vi "License Activator.vi"(8 "error constant":errorcluster) -> (0 "error out":errorcluster)   [LabVIEW 2019]
panel:
  out "Iso Activated":bool
  out "UCT Activated":bool
  out "Sat Activated":bool
  out "Consol Activated":bool
  out "Permea Activated":bool
  out "Shear Activated":bool
  out "TUU Activated":bool
  out "TS Activated":bool
  in  "Iso Generate":bool
  in  "UCT Generate":bool
  in  "Sat Generate":bool
  in  "Cons Generate":bool
  in  "Permeability Generate":bool
  in  "Shearbox Generate":bool
  in  "TUU Generate":bool
  in  "TS Generate":bool
  in  "Isotropic Consolidation":string
  in  "UCT":string
  in  "Saturation (Incremental)":string
  in  "Consolidation (Stepped Loadning/Swelling)":string
  in  "Permeability":string
  in  "Shearbox":string
  in  "Triaxial UU":string
  in  "Triaxial Shear":string
  # "Test Type Module"
  # "Activation Code"
  # "Action"
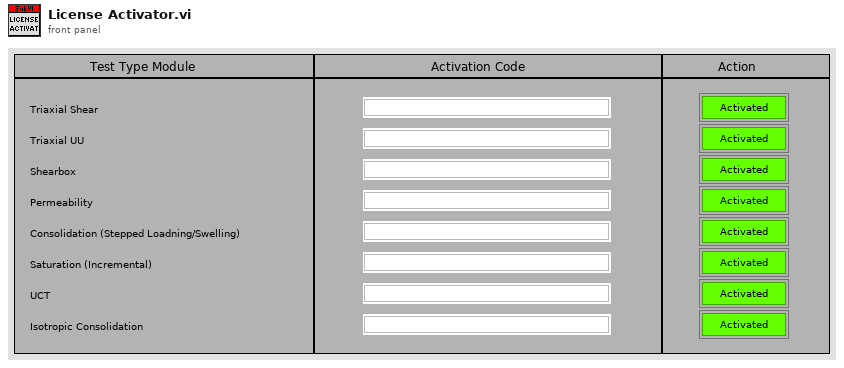
[diagram p1: front panel]
types:
  T1 = enum16{"open", "replace", "create", "open or create", "replace or create", "replace or create with confirmation"}
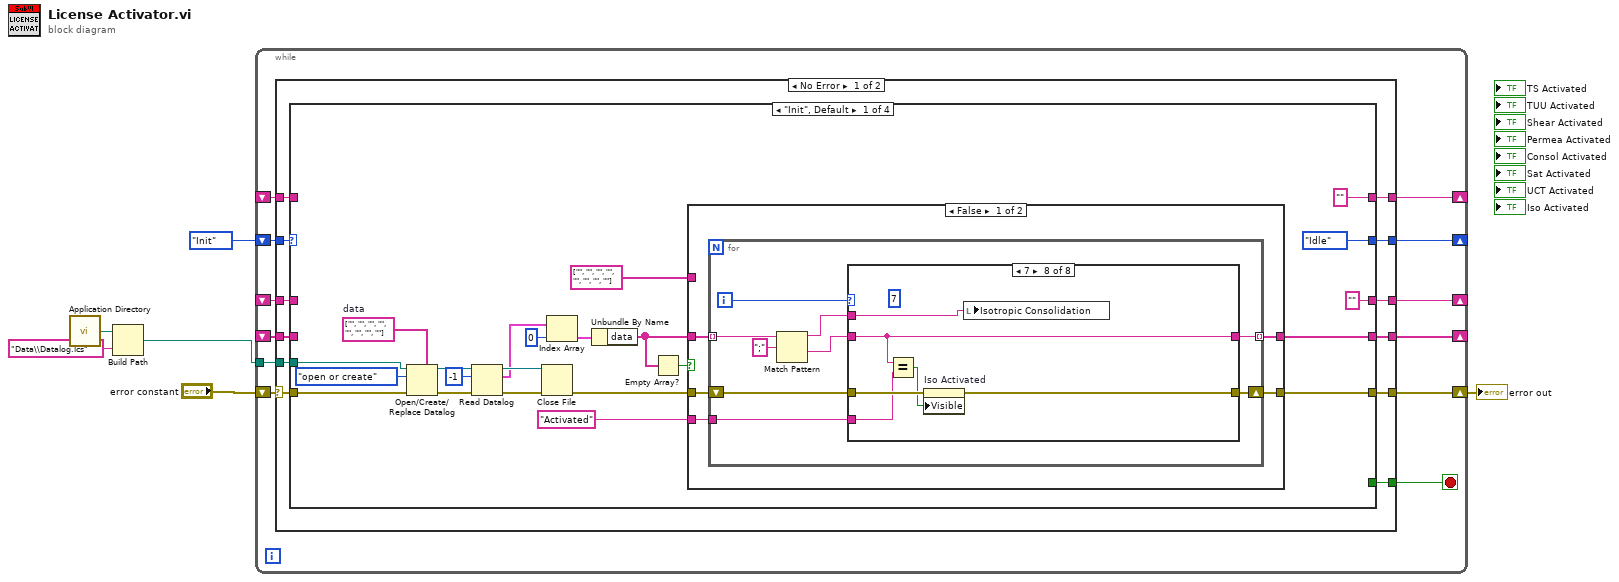
[diagram p0: block diagram]
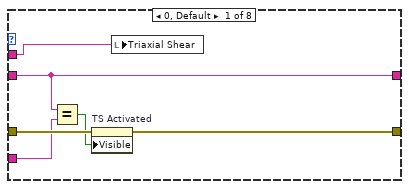
[diagram p2: hidden frame]
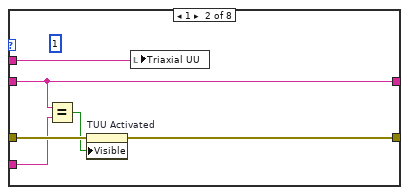
[diagram p3: hidden frame]
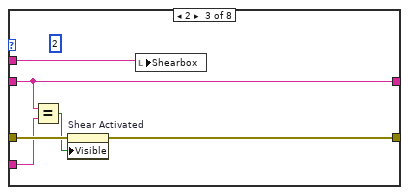
[diagram p4: hidden frame]
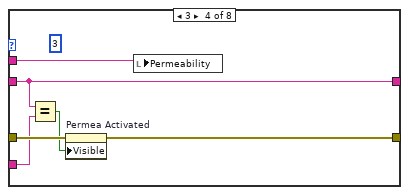
[diagram p5: hidden frame]
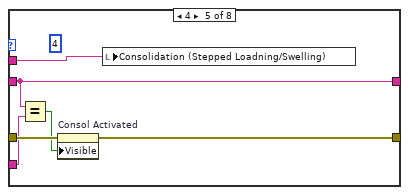
[diagram p6: hidden frame]
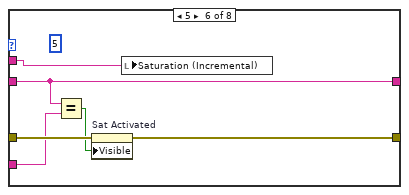
[diagram p7: hidden frame]
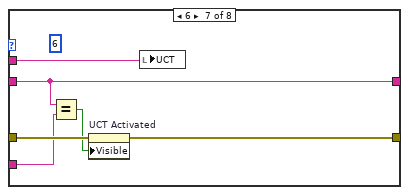
[diagram p8: hidden frame]
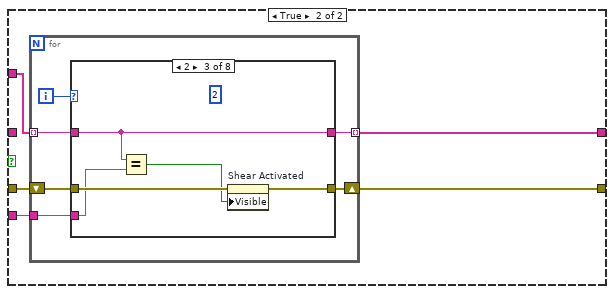
[diagram p9: hidden frame]
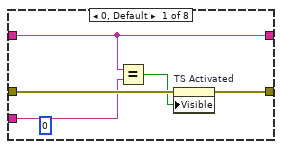
[diagram p10: hidden frame]
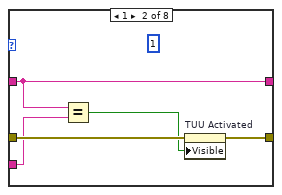
[diagram p11: hidden frame]
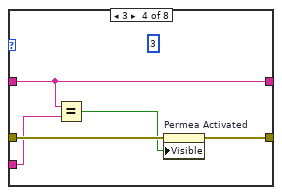
[diagram p12: hidden frame]
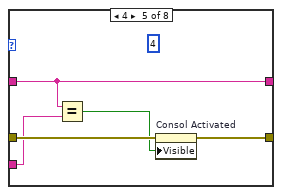
[diagram p13: hidden frame]
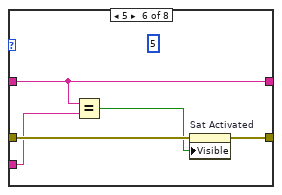
[diagram p14: hidden frame]
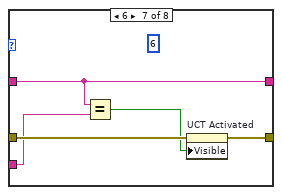
[diagram p15: hidden frame]
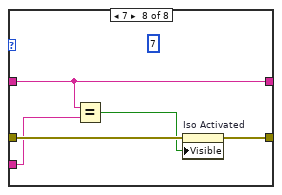
[diagram p16: hidden frame]
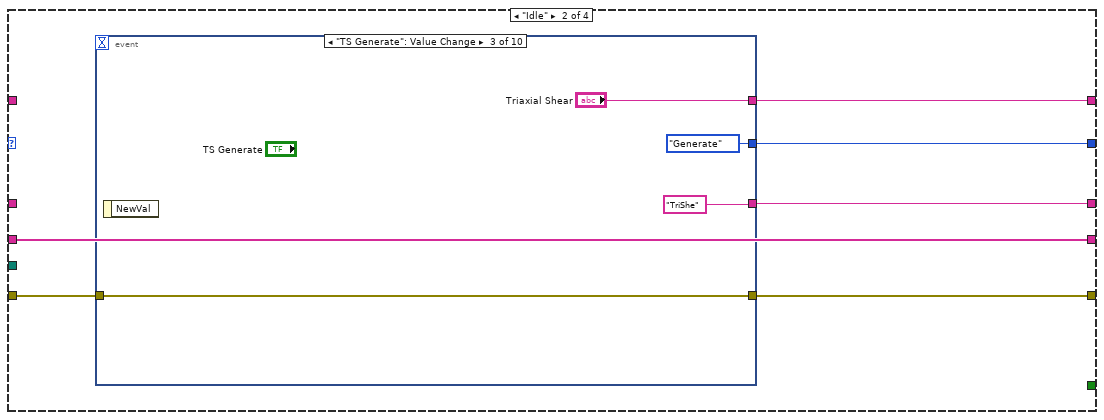
[diagram p17: hidden frame]
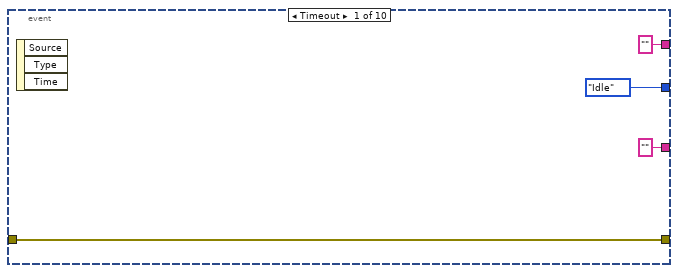
[diagram p18: hidden frame]
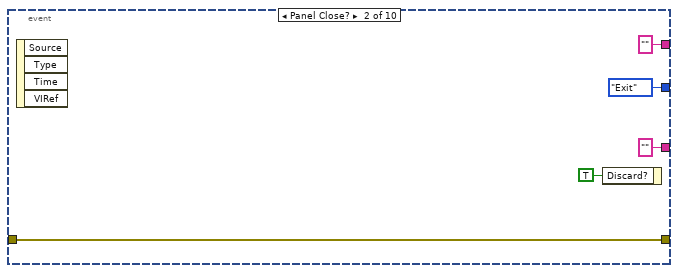
[diagram p19: hidden frame]
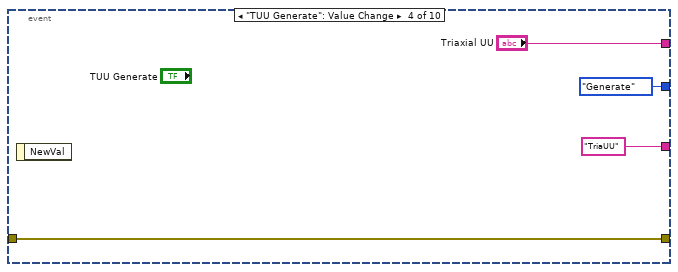
[diagram p20: hidden frame]
diagram:
  n1 = call <vilib>:"Application Directory.vi"() -> ("Application Directory"=w4:path)
  n2 = Build Path(base path=w4, name or relative path="Data\\Datalog.lcs") -> (appended path=w2:path)
  n3 = while {
    shift-right: [w15] -> _
    shift-left: enum16{"Init", "Idle", "Generate", "Exit"}."Init" -> [w18]
    shift-right: [w16] -> w1
    shift-left: "error constant" -> [w17]
    shift-right: [w14] -> _
    shift-left: _ -> [w13]
    shift-right: [w11] -> _
    shift-left: _ -> [w10]
    shift-right: [w9] -> _
    shift-left: _ -> [w8]
    tunnel: w2 -> [w7]
    stop <- w12 stop-if-true
    n4 = case shown="No Error" w17 {
      selector: w17 -> [w28 w291]
      tunnel: w18 -> [w30 _]
      tunnel: [w29 w290] -> w16
      tunnel: [w27 enum16{"Init", "Idle", "Generate", "Exit"}."Idle"] -> w15
      tunnel: [w26 ""] -> w14
      tunnel: w13 -> [w25 _]
      tunnel: [w24 _] -> w12
      tunnel: [w23 ""] -> w11
      tunnel: w10 -> [w22 _]
      tunnel: [w21 w285] -> w9
      tunnel: w8 -> [w20 w285]
      tunnel: w7 -> [w19 _]
      frame No Error {
        n5 = case shown="\"Init\", Default" w30 {
          tunnel: [w37 w171 w233 w284] -> w29
          tunnel: w28 -> [w43 w170 w237 w284]
          tunnel: [enum16{"Init", "Idle", "Generate", "Exit"}."Idle" w169 enum16{"Init", "Idle", "Generate", "Exit"}."Idle" enum16{"Init", "Idle", "Generate", "Exit"}."Exit"] -> w27
          tunnel: ["" w168 "" ""] -> w26
          tunnel: w25 -> [_ _ w215 _]
          tunnel: [_ _ _ TRUE] -> w24
          tunnel: ["" w167 "" ""] -> w23
          tunnel: w22 -> [_ _ w222 _]
          tunnel: [w36 w166 w226 string[] [] ("data")] -> w21
          tunnel: w20 -> [_ w166 w228 _]
          tunnel: w19 -> [w34 _ w225 _]
          frame "Init", Default {
            w47 = string[] ["", "", "", "", "", "", "", ""]  # data
            n6 = Open/Create/Replace Datalog(5:w47, 8:w43, 10:T1."open or create" ("operation (0:open)"), 11:w34) -> (0:w49:errorcluster, 3:w46:refnum<k1>)  [unwired: 2 in, 1 out]
            n7 = Read Datalog(4:w49, 6:-1 ("count (1)"), 7:w46) -> (0:w48:errorcluster, 2:w41:cluster{"data":string[]}[], 3:w45:refnum<k1>)
            n8 = Close File(refnum=w45, error in=w48) -> (error out=w38:errorcluster)  [unwired: 1 out]
            n9 = Index Array(array=w41, index=0) -> (element=w39:cluster{"data":string[]})
            n10 = Unbundle By Name(w39) -> ("data"=w33:string[])
            n11 = Empty Array?(array=w33) -> (empty?=w32:bool)
            n12 = case shown="False" w32 {
              tunnel: w38 -> [w57 w119]
              tunnel: [w56 w118] -> w37
              tunnel: [w55 w117] -> w36
              tunnel: w33 -> [w54 _]
              tunnel: "Activated" ("new element/subarray") -> [w53 w116]
              tunnel: string[] ["", "", "", "", "", "", "", ""] -> [_ w115]
              frame False {
                n13 = for {
                  tunnel: [w64] -> w55 mode=indexing
                  tunnel: w54 -> [w59] mode=indexing
                  tunnel: w53 -> [w63]
                  shift-right: [w65] -> w56
                  shift-left: w57 -> [w66]
                  i -> [w62]
                  n14 = Match Pattern(string=w59, regular expression=";") -> (before substring=w58:string, after substring=w60:string)  [unwired: 1 in, 2 out]
                  n15 = case shown="7" w62 {
                    tunnel: w66 -> [w71 w78 w84 w90 w96 w102 w108 w114]
                    tunnel: [w72 w77 w83 w89 w95 w101 w107 w113] -> w65
                    tunnel: [w68 w74 w81 w87 w94 w100 w106 w112] -> w64
                    tunnel: w60 -> [w68 w74 w81 w87 w94 w100 w106 w112]
                    tunnel: w63 -> [w70 w76 w82 w88 w93 w99 w105 w111]
                    tunnel: w58 -> [w67 w73 w79 w85 w91 w97 w103 w109]
                    frame 0, Default {
                      n16 = Equal?(x=w68, y=w70) -> (x = y?=w69:bool)
                      n17 = property on="TS Activated" class="Bool (strict)"(error in=w71, "Visible"=w69) -> (error out=w72:errorcluster)  [unwired: 1 in, 1 out]
                      n18 = local write "Triaxial Shear"(w67) -> ()
                    }
                    frame 1 {
                      (unwired) 1
                      n19 = Equal?(x=w74, y=w76) -> (x = y?=w75:bool)
                      n20 = property on="TUU Activated" class="Bool (strict)"(error in=w78, "Visible"=w75) -> (error out=w77:errorcluster)  [unwired: 1 in, 1 out]
                      n21 = local write "Triaxial UU"(w73) -> ()
                    }
                    frame 2 {
                      (unwired) 2
                      n22 = Equal?(x=w81, y=w82) -> (x = y?=w80:bool)
                      n23 = property on="Shear Activated" class="Bool (strict)"(error in=w84, "Visible"=w80) -> (error out=w83:errorcluster)  [unwired: 1 in, 1 out]
                      n24 = local write "Shearbox"(w79) -> ()
                    }
                    frame 3 {
                      (unwired) 3
                      n25 = Equal?(x=w87, y=w88) -> (x = y?=w86:bool)
                      n26 = property on="Permea Activated" class="Bool (strict)"(error in=w90, "Visible"=w86) -> (error out=w89:errorcluster)  [unwired: 1 in, 1 out]
                      n27 = local write "Permeability"(w85) -> ()
                    }
                    frame 4 {
                      (unwired) 4
                      n28 = Equal?(x=w94, y=w93) -> (x = y?=w92:bool)
                      n29 = property on="Consol Activated" class="Bool (strict)"(error in=w96, "Visible"=w92) -> (error out=w95:errorcluster)  [unwired: 1 in, 1 out]
                      n30 = local write "Consolidation (Stepped Loadning/Swelling)"(w91) -> ()
                    }
                    frame 5 {
                      (unwired) 5
                      n31 = Equal?(x=w100, y=w99) -> (x = y?=w98:bool)
                      n32 = property on="Sat Activated" class="Bool (strict)"(error in=w102, "Visible"=w98) -> (error out=w101:errorcluster)  [unwired: 1 in, 1 out]
                      n33 = local write "Saturation (Incremental)"(w97) -> ()
                    }
                    frame 6 {
                      (unwired) 6
                      n34 = Equal?(x=w106, y=w105) -> (x = y?=w104:bool)
                      n35 = property on="UCT Activated" class="Bool (strict)"(error in=w108, "Visible"=w104) -> (error out=w107:errorcluster)  [unwired: 1 in, 1 out]
                      n36 = local write "UCT"(w103) -> ()
                    }
                    frame 7 {
                      (unwired) 7
                      n37 = Equal?(x=w112, y=w111) -> (x = y?=w110:bool)
                      n38 = property on="Iso Activated" class="Bool (strict)"(error in=w114, "Visible"=w110) -> (error out=w113:errorcluster)  [unwired: 1 in, 1 out]
                      n39 = local write "Isotropic Consolidation"(w109) -> ()
                    }
                  }
                }
              }
              frame True {
                n40 = for {
                  tunnel: [w123] -> w117 mode=indexing
                  tunnel: w115 -> [w122] mode=indexing
                  tunnel: w116 -> [w121]
                  shift-right: [w124] -> w118
                  shift-left: w119 -> [w125]
                  i -> [w120]
                  n41 = case shown="2" w120 {
                    tunnel: w125 -> [w129 w135 w140 w145 w150 w155 w160 w165]
                    tunnel: [w130 w134 w139 w144 w149 w154 w159 w164] -> w124
                    tunnel: [w126 w131 w137 w142 w148 w153 w158 w163] -> w123
                    tunnel: w122 -> [w126 w131 w137 w142 w148 w153 w158 w163]
                    tunnel: w121 -> [w128 w133 w138 w143 w147 w152 w157 w162]
                    frame 0, Default {
                      (unwired) 0
                      n42 = Equal?(x=w126, y=w128) -> (x = y?=w127:bool)
                      n43 = property on="TS Activated" class="Bool (strict)"(error in=w129, "Visible"=w127) -> (error out=w130:errorcluster)  [unwired: 1 in, 1 out]
                    }
                    frame 1 {
                      (unwired) 1
                      n44 = Equal?(x=w131, y=w133) -> (x = y?=w132:bool)
                      n45 = property on="TUU Activated" class="Bool (strict)"(error in=w135, "Visible"=w132) -> (error out=w134:errorcluster)  [unwired: 1 in, 1 out]
                    }
                    frame 2 {
                      (unwired) 2
                      n46 = Equal?(x=w137, y=w138) -> (x = y?=w136:bool)
                      n47 = property on="Shear Activated" class="Bool (strict)"(error in=w140, "Visible"=w136) -> (error out=w139:errorcluster)  [unwired: 1 in, 1 out]
                    }
                    frame 3 {
                      (unwired) 3
                      n48 = Equal?(x=w142, y=w143) -> (x = y?=w141:bool)
                      n49 = property on="Permea Activated" class="Bool (strict)"(error in=w145, "Visible"=w141) -> (error out=w144:errorcluster)  [unwired: 1 in, 1 out]
                    }
                    frame 4 {
                      (unwired) 4
                      n50 = Equal?(x=w148, y=w147) -> (x = y?=w146:bool)
                      n51 = property on="Consol Activated" class="Bool (strict)"(error in=w150, "Visible"=w146) -> (error out=w149:errorcluster)  [unwired: 1 in, 1 out]
                    }
                    frame 5 {
                      (unwired) 5
                      n52 = Equal?(x=w153, y=w152) -> (x = y?=w151:bool)
                      n53 = property on="Sat Activated" class="Bool (strict)"(error in=w155, "Visible"=w151) -> (error out=w154:errorcluster)  [unwired: 1 in, 1 out]
                    }
                    frame 6 {
                      (unwired) 6
                      n54 = Equal?(x=w158, y=w157) -> (x = y?=w156:bool)
                      n55 = property on="UCT Activated" class="Bool (strict)"(error in=w160, "Visible"=w156) -> (error out=w159:errorcluster)  [unwired: 1 in, 1 out]
                    }
                    frame 7 {
                      (unwired) 7
                      n56 = Equal?(x=w163, y=w162) -> (x = y?=w161:bool)
                      n57 = property on="Iso Activated" class="Bool (strict)"(error in=w165, "Visible"=w161) -> (error out=w164:errorcluster)  [unwired: 1 in, 1 out]
                    }
                  }
                }
              }
            }
          }
          frame "Idle" {
            n58 = event shown="[2] \"TS Generate\": Value Change" {
              selector: _ -> [_ _ _ _ _ _ _ _ _ _]
              dyn-events: _ -> [_ _ _ _ _ _ _ _ _ _]
              timeout: _ -> [_ _ _ _ _ _ _ _ _ _]
              tunnel: [w175 w180 w184 w188 w192 w196 w200 w204 w208 w212] -> w171
              tunnel: w170 -> [w175 w180 w184 w188 w192 w196 w200 w204 w208 w212]
              tunnel: [enum16{"Init", "Idle", "Generate", "Exit"}."Idle" enum16{"Init", "Idle", "Generate", "Exit"}."Exit" enum16{"Init", "Idle", "Generate", "Exit"}."Generate" enum16{"Init", "Idle", "Generate", "Exit"}."Generate" enum16{"Init", "Idle", "Generate", "Exit"}."Generate" enum16{"Init", "Idle", "Generate", "Exit"}."Generate" enum16{"Init", "Idle", "Generate", "Exit"}."Generate" enum16{"Init", "Idle", "Generate", "Exit"}."Generate" enum16{"Init", "Idle", "Generate", "Exit"}."Generate" enum16{"Init", "Idle", "Generate", "Exit"}."Generate"] -> w169
              tunnel: ["" "" "Triaxial Shear" "Triaxial UU" "Shearbox" "Permeability" "Consolidation (Stepped Loadning/Swelling)" "Saturation (Incremental)" "UCT" "Isotropic Consolidation"] -> w168
              tunnel: ["" "" "TriShe" "TriaUU" "Shearb" "Permea" "Consol" "Satura" "UCTUCT" "IsoCon"] -> w167
              event Timeout {
                n59 = event-data() -> ()  [unwired: 1 in, 3 out]
              }
              event Panel Close? {
                n60 = event-data() -> ()  [unwired: 1 in, 4 out]
                n61 = event-data("Discard?"=TRUE) -> ()  [unwired: 1 in, 1 out]
              }
              event "TS Generate": Value Change {
                n62 = event-data() -> ()  [unwired: 1 in, 1 out]
              }
              event "TUU Generate": Value Change {
                n63 = event-data() -> ()  [unwired: 1 in, 1 out]
              }
              event "Shearbox Generate": Value Change {
                n64 = event-data() -> ()  [unwired: 1 in, 1 out]
              }
              event "Permeability Generate": Value Change {
                n65 = event-data() -> ()  [unwired: 1 in, 1 out]
              }
              event "Cons Generate": Value Change {
                n66 = event-data() -> ()  [unwired: 1 in, 1 out]
              }
              event "Sat Generate": Value Change {
                n67 = event-data() -> ()  [unwired: 1 in, 1 out]
              }
              event "UCT Generate": Value Change {
                n68 = event-data() -> ()  [unwired: 1 in, 1 out]
              }
              event "Iso Generate": Value Change {
                n69 = event-data() -> ()  [unwired: 1 in, 1 out]
              }
            }
          }
          frame "Generate" {
            n70 = call "Main - Decrypt (SubVI).vi"("Base64 String"=w215) -> ("String"=w224:string)  [unwired: 9 in]
            n71 = String To Byte Array(string=w222) -> (unsigned byte array=w221:u8[])
            n72 = String To Byte Array(string=w224) -> (unsigned byte array=w223:u8[])
            n73 = for {
              tunnel: w223 -> [w244]
              tunnel: w221 -> [w243] mode=indexing
              tunnel: [w241] -> w220 mode=indexing
              n74 = Search 1D Array(1D array=w244, element=w243) -> (index of element=w242:i32)  [unwired: 1 in]
              n75 = Greater Or Equal To 0?(x=w242) -> (x >= 0?=w241:bool)
            }
            n76 = And Array Elements(Boolean array=w220) -> (logical AND=w218:bool)
            n77 = case shown="\"Permea\"" w222 {
              tunnel: w218 -> [_ w248 w252 w256 w260 w264 w268 w272 w276]
              tunnel: w237 -> [w246 w249 w254 w258 w262 w266 w270 w274 w278]
              tunnel: [w246 w250 w253 w257 w261 w265 w269 w273 w277] -> w234
              tunnel: [-1 0 1 2 3 4 5 6 7] -> w227
              frame Default {
              }
              frame "TriShe" {
                n78 = property on="TS Activated" class="Bool (strict)"(error in=w249, "Visible"=w248) -> (error out=w250:errorcluster)  [unwired: 1 in, 1 out]
              }
              frame "TriaUU" {
                n79 = property on="TUU Activated" class="Bool (strict)"(error in=w254, "Visible"=w252) -> (error out=w253:errorcluster)  [unwired: 1 in, 1 out]
              }
              frame "Shearb" {
                n80 = property on="Shear Activated" class="Bool (strict)"(error in=w258, "Visible"=w256) -> (error out=w257:errorcluster)  [unwired: 1 in, 1 out]
              }
              frame "Permea" {
                n81 = property on="Permea Activated" class="Bool (strict)"(error in=w262, "Visible"=w260) -> (error out=w261:errorcluster)  [unwired: 1 in, 1 out]
              }
              frame "Consol" {
                n82 = property on="Consol Activated" class="Bool (strict)"(error in=w266, "Visible"=w264) -> (error out=w265:errorcluster)  [unwired: 1 in, 1 out]
              }
              frame "Satura" {
                n83 = property on="Sat Activated" class="Bool (strict)"(error in=w270, "Visible"=w268) -> (error out=w269:errorcluster)  [unwired: 1 in, 1 out]
              }
              frame "UCTUCT" {
                n84 = property on="UCT Activated" class="Bool (strict)"(error in=w274, "Visible"=w272) -> (error out=w273:errorcluster)  [unwired: 1 in, 1 out]
              }
              frame "IsoCon" {
                n85 = property on="Iso Activated" class="Bool (strict)"(error in=w278, "Visible"=w276) -> (error out=w277:errorcluster)  [unwired: 1 in, 1 out]
              }
            }
            n86 = Concatenate Strings(w215, ";" ("string"), "Activated" ("new element/subarray")) -> (w213:string)
            n87 = Select(t=w213, s=w218, f="") -> (s? t:f=w219:string)
            n88 = Replace Array Subset(array=w228, new element=w219, index=w227) -> (w226:string[])
            n89 = Open/Create/Replace Datalog(5:string[] ["", "", "", "", "", "", "", ""], 8:w234, 10:T1."replace or create" ("operation (0:open)"), 11:w225) -> (0:w236:errorcluster, 3:w231:refnum<k1>)  [unwired: 2 in, 1 out]
            n90 = Write Datalog(4:w236, 6:w226, 7:w231) -> (0:w235:errorcluster, 3:w230:refnum<k1>)
            n91 = Close File(refnum=w230, error in=w235) -> (error out=w233:errorcluster)  [unwired: 1 out]
          }
          frame "Exit" {
          }
        }
      }
      frame Error {
        n92 = call <vilib>:"Clear Errors.vi"("error in (no error)"=w291) -> ("error out"=w290:errorcluster)  [unwired: 5 in, 1 out]
        n93 = Wait (ms)(milliseconds to wait=u32 100) -> ()  [unwired: 1 out]
      }
    }
  }
  "error out" <- w1
